vi "Dynamic Graphs.vi"() -> ()   [LabVIEW 2024]
panel:
  in  "stop":bool
  out "XY Graph":cluster{i32[], i32[]}(graph)
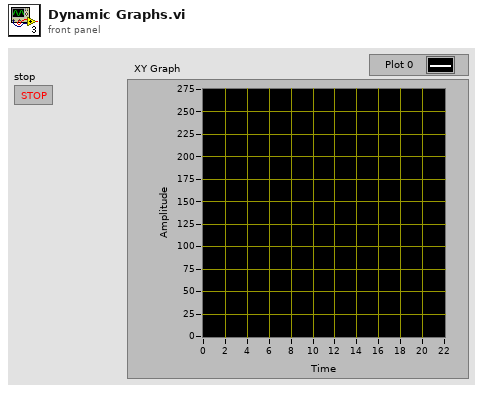
[diagram p1: front panel]
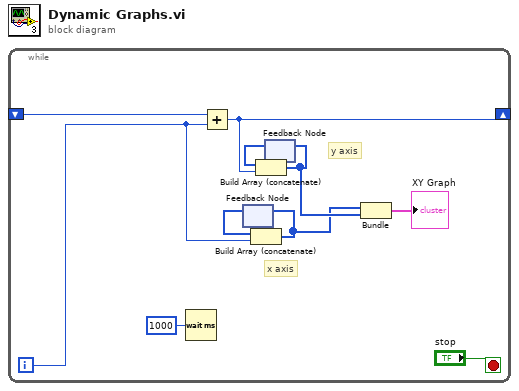
[diagram p0: block diagram]
diagram:
  n1 = while {
    shift-right: [w8] -> _
    shift-left: _ -> [w9]
    i -> [w6]
    stop <- "stop" stop-if-true
    # "x axis"
    # "y axis"
    n2 = Wait (ms)(milliseconds to wait=u32 1000) -> ()  [unwired: 1 out]
    n3 = Add(x=w9, y=w6) -> (x+y=w8:i32)
    n4 = feedback #1() -> (w5:i32[])  [unwired: 1 in]
    n5 = Build Array (concatenate)(w5, w6) -> (w3:i32[])
    n6 = feedback-in #1(w3) -> ()
    n7 = feedback #2() -> (w7:i32[])  [unwired: 1 in]
    n8 = Build Array (concatenate)(w7, w8) -> (w4:i32[])
    n9 = feedback-in #2(w4) -> ()
    n10 = Bundle(w3, w4) -> (→"XY Graph":cluster{i32[], i32[]})  [unwired: 1 in]
  }
